vi "Obtain Priority Queue.vi"(8 "error in (no error)":errorcluster, 9 "create if not found? (T)":bool=TRUE, 11 "name":string) -> (0 "error out":errorcluster, 1 "created new?":bool, 3 "Priority Queue":refnum<class "Priority Queue.lvclass">)   [LabVIEW 2020, in "Communicable State Machine.lvlib" / "Priority Queue.lvclass"]
uses:
  Priority Queue.lvclass
  _Cross CSM State Data.ctl
  _CSM_MSG_TYPE.ctl
  _Cross CSM State Response.ctl
  _CSM_Response Source Message.ctl
  def-Data(LowPRI-Q).ctl
  Priority Queue.lvclass/Priority Queue.ctl
  Communicable State Machine.lvlib
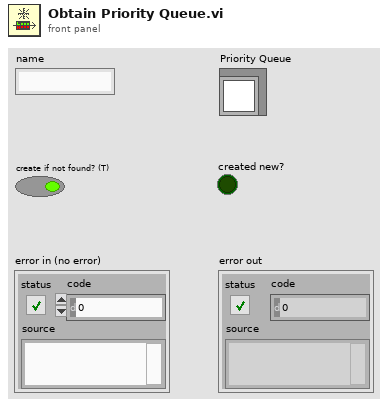
[diagram p1: front panel]
types:
  T1 = typedef "Communicable State Machine.lvlib/_Cross CSM State Data.ctl" = cluster{"Msg Type":T2, "state":string, "args":string, "source":string, "RespQ":refnum<queue>, "Response For Message":T3, "Target":string}
  T2 = typedef "Communicable State Machine.lvlib/_CSM_MSG_TYPE.ctl" = enum16{"Sync Message(-@)", "Async Message(->)", "Async without Response(->|)", "Async Response", "Broadcast(-><all>)", "Broadcast(-><status>)", "Broadcast(-><interrupt>)", "Append to JKISM States", "Append to JKISM States(High Priority)"}
  T3 = typedef "Communicable State Machine.lvlib/_CSM_Response Source Message.ctl" = cluster{"‘State":string, "’Arguments":string, "’Error":errorcluster}
  T4 = typedef "Communicable State Machine.lvlib/Priority Queue.lvclass/def-Data(LowPRI-Q).ctl" = cluster{"Data":T1, "Notify?":bool}
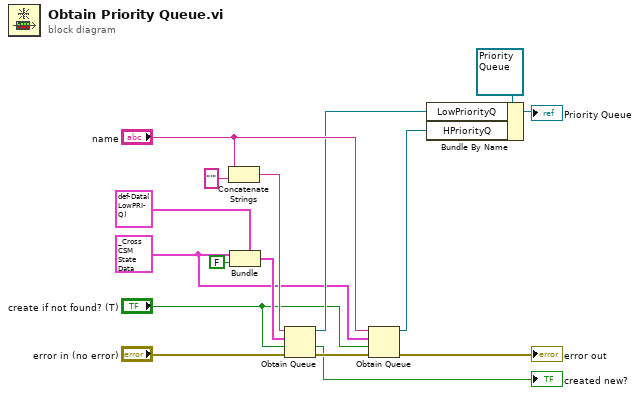
[diagram p0: block diagram]
diagram:
  w3 = T1 {"Msg Type"=enum."Sync Message(-@)", "state"="", "args"="", "source"="", "RespQ"=refnum, "Response For Message"={"‘State"="", "’Arguments"="", "’Error"={"status"=FALSE, "code"=0, "source"=""}}, "Target"=""} ("Cross JKI State Machine State")
  n1 = Concatenate Strings("name", "'" ("string")) -> (w15:string)
  n2 = Bundle(cluster=T4 {"Data"={"Msg Type"=enum."Sync Message(-@)", "state"="", "args"="", "source"="", "RespQ"=refnum, "Response For Message"={"‘State"="", "’Arguments"="", "’Error"={"status"=FALSE, "code"=0, "source"=""}}, "Target"=""}, "Notify?"=FALSE}, "Data"=w3, "Notify?"=FALSE) -> (w8:T4)
  n3 = Obtain Queue(name (unnamed)=w15, element data type=w8, create if not found? (T)="create if not found? (T)", error in (no error)="error in (no error)") -> (queue out=w10:refnum<queue>, created new?=→"created new?":bool, error out=w6:errorcluster)  [unwired: 1 in]
  n4 = Obtain Queue(name (unnamed)="name", element data type=w3, create if not found? (T)="create if not found? (T)", error in (no error)=w6) -> (queue out=w1:refnum<queue>, error out=→"error out":errorcluster)  [unwired: 1 in, 1 out]
  n5 = Bundle By Name(cluster=refnum<class "Priority Queue.lvclass"> refnum ("Priority Queue"), "LowPriorityQ"=w10, "HPriorityQ"=w1) -> (→"Priority Queue":refnum<class "Priority Queue.lvclass">)
